vi "Initiate Stream.vi"(0 "Register Bus":T1, 1 "scope":string(combo)="rx", 11 "error in":errorcluster) -> (4 "Register Bus (out)":T1, 15 "error out":errorcluster)   [LabVIEW 2017]
doc: "Initiate the stream. This is required before acquiring/generating data with the Fetch Rx Data or Write Tx Data VIs. Initiation includes resetting the rx/tx streams and the DSP.\n\n<B>Input Parameters</B>\n\n<B>Register Bus</B> The Register Bus object created by the ni579x Open VI and used as the session handle for the NI-579x Configuration Design Library.\n\n<B>scope</B> is the channel to initiate the stream for. The options are \"rx\" and \"tx\".\n\n<B>error in</B> describes error conditions that occur before this node runs. This input provides standard 'error in' functionality.\n\n<B>Output Parameters</B>\n\n<B>Register Bus (out)</B> The Register Bus object created by the ni579x Open VI and used as the session handle for the NI-579x Configuration Design Library.\n\n<B>error out</B> contains error information. This output provides standard 'error out' functionality."
uses:
  <instrlib>/_niInstr/Register Bus/v0/Host/Public/Register Bus Session.ctl
  <instrlib>/_niInstr/Register Bus/v0/Host/Private/Session Data.ctl
  Tx FPGA VI Reference.ctl
  Rx FPGA VI Reference.ctl
  <vilib>/Utility/error.llb/Error Cluster From Error Code.vi
  <vilib>/rvi/errors/niLvFpgaAdjustHostInterfaceError.vi
  <vilib>/ErrorRing/Error Ring.xnode
  <vilib>/rvi/interface/nirviReadWriteControl/nirviReadWriteControl.xnode
  <vilib>/rvi/interface/Simulation/niFpgaSimulationCallBeginRW.vi
  NiFpgaLv.dll
  <instrlib>/_niInstr/Register Bus/v0/Host/niInstr Register Bus v0 Host.lvlib
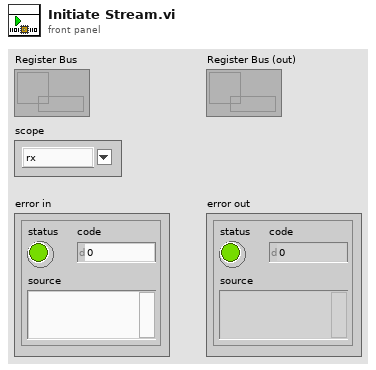
[diagram p1: front panel]
types:
  T1 = typedef "niInstr Register Bus v0 Host.lvlib/Register Bus Session.ctl" = refnum<queue>
  T2 = typedef "Tx FPGA VI Reference.ctl" = refnum<k20>
  T3 = typedef "Rx FPGA VI Reference.ctl" = refnum<k20>
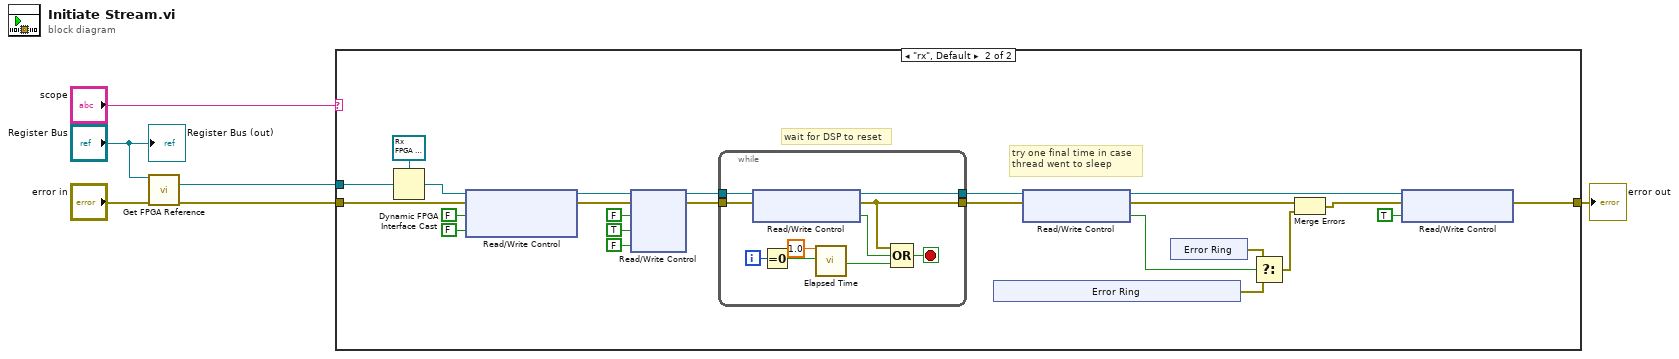
[diagram p0: block diagram]
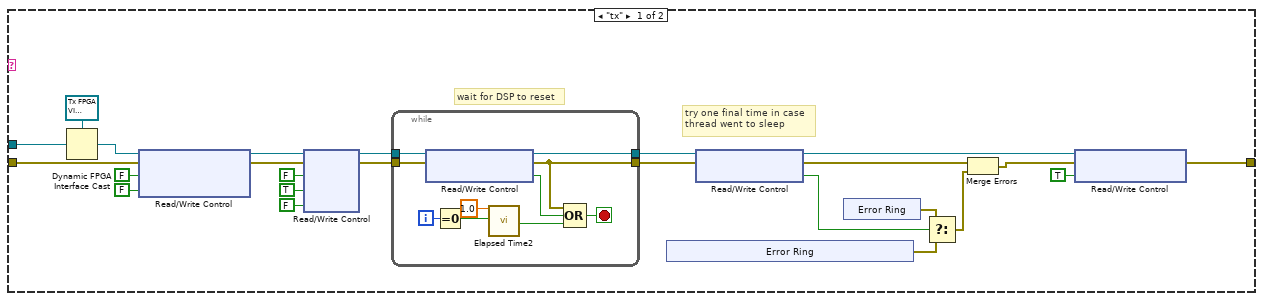
[diagram p2: hidden frame]
diagram:
  n1 = call <instrlib>:"Get FPGA Reference.vi"("session in"="Register Bus", "error in"="error in") -> ("fpga ref"=w4:refnum<k20>, "error out"=w2:errorcluster)  [unwired: 11 in, 1 out]
  n2 = case shown="\"rx\", Default" "scope" {
    tunnel: w4 -> [w20 w70]
    tunnel: [w18 w59] -> w3
    tunnel: w2 -> [w19 w53]
    frame "tx" {
      # "try one final time in case\nthread went to sleep"
      # "wait for DSP to reset"
      n3 = Dynamic FPGA Interface Cast(Session In=T2 refnum ("FPGA VI Reference Out"), Type=w20) -> (Session Out=w23:T2)
      n4 = xnode "Read/Write Control"("FPGA VI Reference In"=w23, "error in"=w19, "tx.stream enabled"=FALSE, "tx.abort"=FALSE) -> ("FPGA VI Reference Out"=w21:T2, "error out"=w22:errorcluster)
      n5 = xnode "Read/Write Control"("FPGA VI Reference In"=w21, "error in"=w22, "tx.reset"=FALSE, "tx.reset"=TRUE, "tx.reset"=FALSE) -> ("FPGA VI Reference Out"=w10:T2, "error out"=w9:errorcluster)
      n6 = while {
        tunnel: w10 -> [w46]
        tunnel: w9 -> [w45]
        tunnel: [w38] -> w17
        tunnel: [w37] -> w16
        i -> [w43]
        stop <- w39 stop-if-true
        n7 = xnode "Read/Write Control"("FPGA VI Reference In"=w46, "error in"=w45) -> ("FPGA VI Reference Out"=w37:T2, "error out"=w38:errorcluster, "tx.dsp reset done"=w41:bool)
        n8 = Equal To 0?(x=w43) -> (x = 0?=w44:bool)
        n9 = call "Elapsed Time2"("Time Target (s)"=1.0, "Reset"=w44) -> ("Time has Elapsed"=w40:bool)  [unwired: 10 in, 7 out]
        n10 = Compound Arithmetic op=OR(w38, w41, w40) -> (w39:bool)
      }
      n11 = xnode "Error Ring"() -> ("error out"=w11:errorcluster)
      n12 = xnode "Read/Write Control"("FPGA VI Reference In"=w16, "error in"=w17) -> ("FPGA VI Reference Out"=w7:T2, "error out"=w14:errorcluster, "tx.dsp reset done"=w15:bool)
      n13 = xnode "Error Ring"() -> ("error out"=w12:errorcluster)
      n14 = Select(t=w12, s=w15, f=w11) -> (s? t:f=w13:errorcluster)
      n15 = Merge Errors(w14, w13) -> (w8:errorcluster)
      n16 = xnode "Read/Write Control"("FPGA VI Reference In"=w7, "error in"=w8, "tx.stream enabled"=TRUE) -> ("error out"=w18:errorcluster)  [unwired: 1 out]
    }
    frame "rx", Default {
      # "try one final time in case\nthread went to sleep"
      # "wait for DSP to reset"
      n17 = Dynamic FPGA Interface Cast(Session In=T3 refnum ("Type"), Type=w70) -> (Session Out=w54:T3)
      n18 = xnode "Read/Write Control"("FPGA VI Reference In"=w54, "error in"=w53, "rx.stream enabled"=FALSE, "rx.abort"=FALSE) -> ("FPGA VI Reference Out"=w51:T3, "error out"=w50:errorcluster)
      n19 = xnode "Read/Write Control"("FPGA VI Reference In"=w51, "error in"=w50, "rx.reset"=FALSE ("Acquisition.Reset"), "rx.reset"=TRUE, "rx.reset"=FALSE) -> ("FPGA VI Reference Out"=w55:T3, "error out"=w56:errorcluster)
      n20 = while {
        tunnel: w55 -> [w86]
        tunnel: w56 -> [w85]
        tunnel: [w78] -> w67
        tunnel: [w77] -> w66
        i -> [w83]
        stop <- w79 stop-if-true
        n21 = xnode "Read/Write Control"("FPGA VI Reference In"=w86, "error in"=w85) -> ("FPGA VI Reference Out"=w77:T3, "error out"=w78:errorcluster, "rx.dsp reset done"=w81:bool)
        n22 = Equal To 0?(x=w83) -> (x = 0?=w84:bool)
        n23 = call "Elapsed Time"("Time Target (s)"=1.0, "Reset"=w84) -> ("Time has Elapsed"=w80:bool)  [unwired: 10 in, 7 out]
        n24 = Compound Arithmetic op=OR(w78, w81, w80) -> (w79:bool)
      }
      n25 = xnode "Error Ring"() -> ("error out"=w61:errorcluster)
      n26 = xnode "Read/Write Control"("FPGA VI Reference In"=w66, "error in"=w67) -> ("FPGA VI Reference Out"=w47:T3, "error out"=w64:errorcluster, "rx.dsp reset done"=w65:bool)
      n27 = xnode "Error Ring"() -> ("error out"=w62:errorcluster)
      n28 = Select(t=w62, s=w65, f=w61) -> (s? t:f=w63:errorcluster)
      n29 = Merge Errors(w64, w63) -> (w48:errorcluster)
      n30 = xnode "Read/Write Control"("FPGA VI Reference In"=w47, "error in"=w48, "rx.stream enabled"=TRUE) -> ("error out"=w59:errorcluster)  [unwired: 1 out]
    }
  }
  "error out" <- w3
  "Register Bus (out)" <- "Register Bus"
